vi "CryoCon_RampControl.vi"() -> ()   [LabVIEW 2026]
panel:
  in  "STOP CONTROL":bool
  in  "Target Setpoint (K)":dbl=273.15
  in  "EXIT":bool
  in  "GO TO SETPOINT":bool
  out "Heater (%)":i32=5
  out "Temperature (K)":dbl format="%.2f"
  out "Input String":string
  in  "VISA resource name":refnum<visa-resource-name>="COM5"
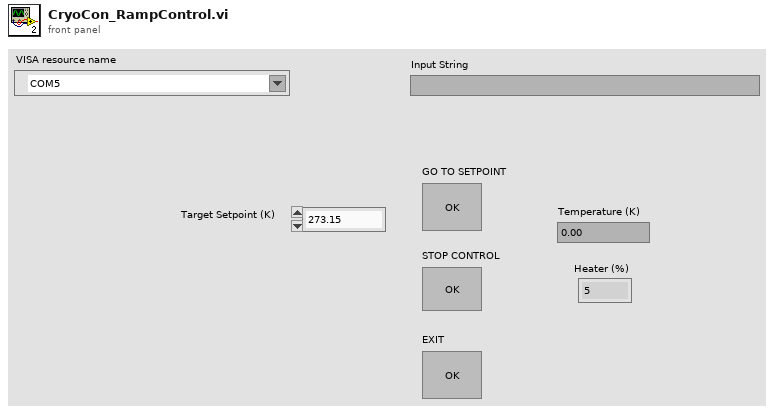
[diagram p1: front panel]
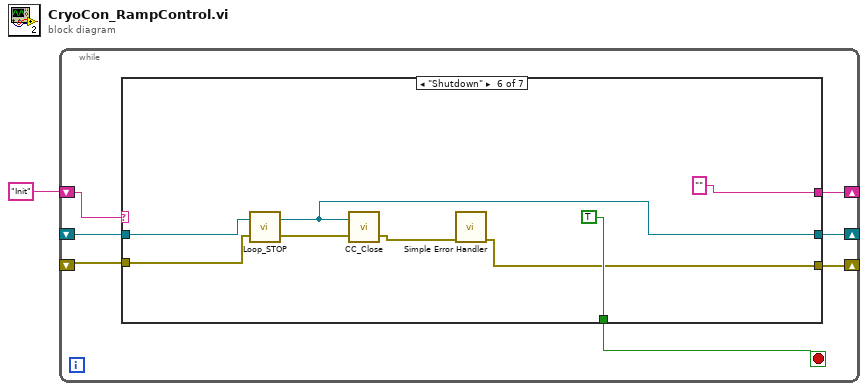
[diagram p0: block diagram]
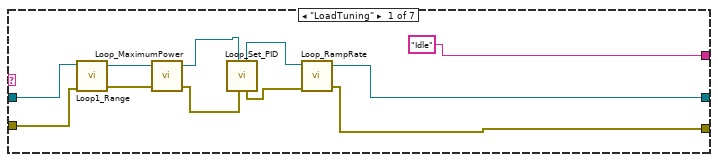
[diagram p2: hidden frame]
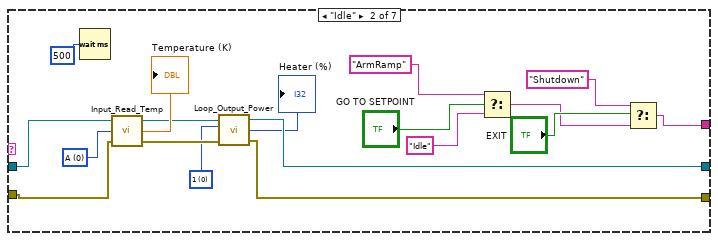
[diagram p3: hidden frame]
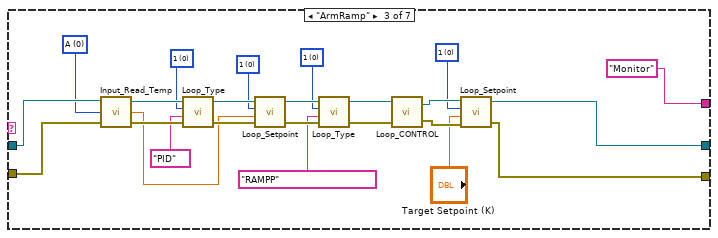
[diagram p4: hidden frame]
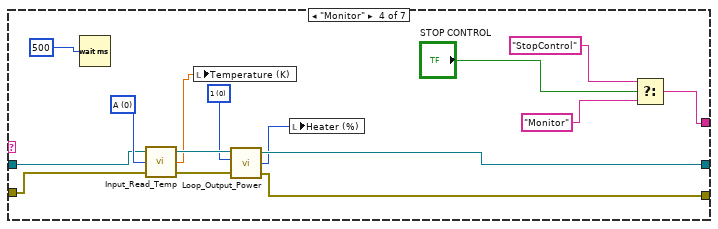
[diagram p5: hidden frame]
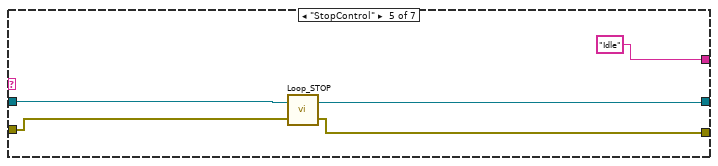
[diagram p6: hidden frame]
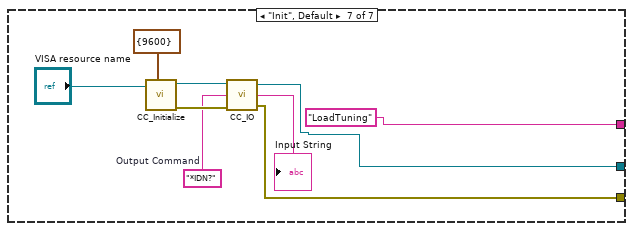
[diagram p7: hidden frame]
diagram:
  n1 = while {
    shift-right: [w5] -> _
    shift-left: "Init" -> [w8]
    shift-right: [w7] -> _
    shift-left: _ -> [w4]
    shift-right: [w6] -> _
    shift-left: _ -> [w3]
    stop <- w2 stop-if-true
    n2 = case shown="\"Shutdown\"" w8 {
      tunnel: [w12 w30 w48 w69 w79 w82 w90] -> w7
      tunnel: [w11 w31 w49 w68 w78 w83 w92] -> w6
      tunnel: ["Idle" w22 "Monitor" w62 "Idle" "" "LoadTuning"] -> w5
      tunnel: w4 -> [w16 w35 w61 w74 w81 w89 _]
      tunnel: w3 -> [w10 w33 w55 w73 w80 w87 _]
      tunnel: [_ _ _ _ _ TRUE _] -> w2
      frame "LoadTuning" {
        n3 = call "Loop1_Range.vi"("VISA in"=w16, "error in"=w10) -> ("VISA out"=w19:refnum<visa-resource-name>, "ErrorOut"=w15:errorcluster)  [unwired: 3 in, 1 out]
        n4 = call "Loop_MaximumPower.vi"("VISA in"=w19, "error in"=w15) -> ("VISA out"=w18:refnum<visa-resource-name>, "ErrorOut"=w14:errorcluster)  [unwired: 3 in, 1 out]
        n5 = call "Loop_Set_PID.vi"("error in (no error)"=w14, "VISA In"=w18) -> ("error out"=w13:errorcluster, "VISA Out"=w17:refnum<visa-resource-name>)  [unwired: 8 in]
        n6 = call "Loop_RampRate.vi"("VISA in"=w17, "error in"=w13) -> ("VISA out"=w12:refnum<visa-resource-name>, "ErrorOut"=w11:errorcluster)  [unwired: 3 in, 1 out]
      }
      frame "Idle" {
        w28 = u8 0 items=["1", "2", "3", "4"] ("Loop")
        w37 = u8 0 items=["A", "B", "C", "D"] ("Input")
        n7 = Wait (ms)(milliseconds to wait=u32 500) -> ()  [unwired: 1 out]
        n8 = call "Input_Read_Temp.vi"("error in (no error)"=w33, "Input"=w37, "VISA In"=w35) -> ("error out"=w32:errorcluster, "Temperature"=→"Temperature (K)":dbl, "VISA Out"=w34:refnum<visa-resource-name>)
        n9 = call "Loop_Output_Power.vi"("VISA in"=w34, "Loop"=w28, "error in"=w32) -> ("VISA out"=w30:refnum<visa-resource-name>, "Output Pwr (%)"=→"Heater (%)":i32, "ErrorOut"=w31:errorcluster)  [unwired: 2 in]
        n10 = Select(t="ArmRamp", s="GO TO SETPOINT", f="Idle") -> (s? t:f=w20:string)
        n11 = Select(t="Shutdown", s="EXIT", f=w20) -> (s? t:f=w22:string)
      }
      frame "ArmRamp" {
        w41 = u8 0 items=["1", "2", "3", "4"] ("Loop")
        w43 = u8 0 items=["1", "2", "3", "4"] ("Loop")
        w44 = u8 0 items=["1", "2", "3", "4"] ("Loop")
        w46 = u8 0 items=["1", "2", "3", "4"] ("Loop")
        w47 = u8 0 items=["A", "B", "C", "D"] ("Input")
        n12 = call "Input_Read_Temp.vi"("error in (no error)"=w55, "Input"=w47, "VISA In"=w61) -> ("error out"=w54:errorcluster, "Temperature"=w38:dbl, "VISA Out"=w60:refnum<visa-resource-name>)
        n13 = call "Loop_Type.vi"("VISA in"=w60, "Loop"=w46, "Loop Type"="PID", "error in"=w54) -> ("VISA out"=w59:refnum<visa-resource-name>, "ErrorOut"=w53:errorcluster)  [unwired: 1 in, 1 out]
        n14 = call "Loop_Setpoint.vi"("VISA in"=w59, "Loop"=w44, "Setpoint"=w38, "error in"=w53) -> ("VISA out"=w58:refnum<visa-resource-name>, "ErrorOut"=w52:errorcluster)  [unwired: 1 in, 1 out]
        n15 = call "Loop_Type.vi"("VISA in"=w58, "Loop"=w43, "Loop Type"="RAMPP", "error in"=w52) -> ("VISA out"=w57:refnum<visa-resource-name>, "ErrorOut"=w51:errorcluster)  [unwired: 1 in, 1 out]
        n16 = call "Loop_CONTROL.vi"("error in (no error)"=w51, "VISA In"=w57) -> ("error out"=w50:errorcluster, "VISA Out"=w56:refnum<visa-resource-name>)
        n17 = call "Loop_Setpoint.vi"("VISA in"=w56, "Loop"=w41, "Setpoint"="Target Setpoint (K)", "error in"=w50) -> ("VISA out"=w48:refnum<visa-resource-name>, "ErrorOut"=w49:errorcluster)  [unwired: 1 in, 1 out]
      }
      frame "Monitor" {
        w70 = u8 0 items=["1", "2", "3", "4"] ("Loop")
        w75 = u8 0 items=["A", "B", "C", "D"] ("Input")
        n18 = Wait (ms)(milliseconds to wait=u32 500) -> ()  [unwired: 1 out]
        n19 = call "Input_Read_Temp.vi"("error in (no error)"=w73, "Input"=w75, "VISA In"=w74) -> ("error out"=w71:errorcluster, "Temperature"=w67:dbl, "VISA Out"=w72:refnum<visa-resource-name>)
        n20 = local write "Temperature (K)"(w67) -> ()
        n21 = call "Loop_Output_Power.vi"("VISA in"=w72, "Loop"=w70, "error in"=w71) -> ("VISA out"=w69:refnum<visa-resource-name>, "Output Pwr (%)"=w66:i32, "ErrorOut"=w68:errorcluster)  [unwired: 2 in]
        n22 = local write "Heater (%)"(w66) -> ()
        n23 = Select(t="StopControl", s="STOP CONTROL", f="Monitor") -> (s? t:f=w62:string)
      }
      frame "StopControl" {
        n24 = call "Loop_STOP.vi"("error in (no error)"=w80, "VISA In"=w81) -> ("error out"=w78:errorcluster, "VISA Out"=w79:refnum<visa-resource-name>)
      }
      frame "Shutdown" {
        n25 = call "Loop_STOP.vi"("error in (no error)"=w87, "VISA In"=w89) -> ("error out"=w86:errorcluster, "VISA Out"=w82:refnum<visa-resource-name>)
        n26 = call "CC_Close.vi"("error in (no error)"=w86, "VISA In"=w82) -> ("error out"=w88:errorcluster)  [unwired: 1 in]
        n27 = call <vilib>:"Simple Error Handler.vi"("error in (no error)"=w88) -> ("error out"=w83:errorcluster)  [unwired: 4 in, 4 out]
      }
      frame "Init", Default {
        w94 = "*IDN?"  # Output Command
        n28 = call "CC_Initialize.vi"("Serial Configuration"=cluster{"Baud Rate":u32} {"Baud Rate"=9600}, "VISA resource name"="VISA resource name") -> ("error out"=w95:errorcluster, "VISA resource name out"=w96:refnum<visa-resource-name>)  [unwired: 8 in]
        n29 = call "CC_IO.vi"("error in (no error)"=w95, "Output Command"=w94, "VISA In"=w96) -> ("error out"=w92:errorcluster, "Input String"=→"Input String":string, "VISA out"=w90:refnum<visa-resource-name>)
      }
    }
  }
